vi "poly_h5_write_array_1d_DBL.vi"(0 "h5 dir ref":i32, 1 "dataset name":string, 5 "array":dbl[](array[numeric]), 7 "units (au)":string="au", 11 "error in (no error)":errorcluster, 12 "dim (index)":string="index") -> (4 "h5 obj ref":i32, 15 "error out":errorcluster)   [LabVIEW 2015]
uses:
  <vilib>/addons/h5labview2/base/lib_path.vi
  <vilib>/addons/h5labview2/base/H5Equery.vi
  <vilib>/addons/h5labview2/dataset/H5Dwrite.llb/H5Dwrite.xnode
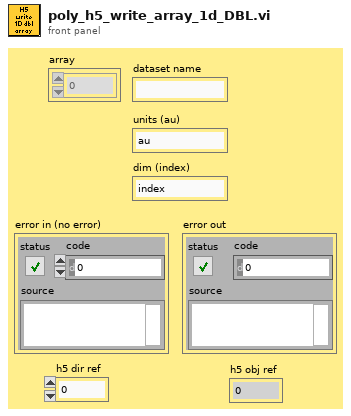
[diagram p1: front panel]
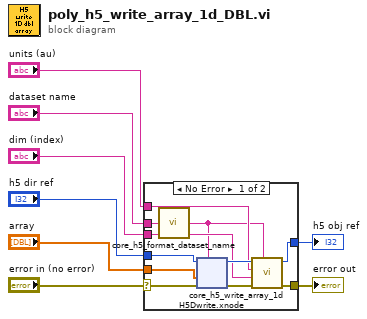
[diagram p0: block diagram]
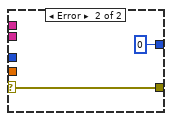
[diagram p2: hidden frame]
diagram:
  n1 = case shown="No Error" "error in (no error)" {
    selector: "error in (no error)" -> [w17 w40]
    tunnel: "h5 dir ref" -> [w19 _]
    tunnel: "array" -> [w18 _]
    tunnel: "dataset name" -> [w10 _]
    tunnel: [w13 w40] -> w6
    tunnel: [w15 0] -> w5
    tunnel: "dim (index)" -> [w12 _]
    tunnel: "units (au)" -> [w11 _]
    frame No Error {
      n2 = call "core_h5_format_dataset_name.vi"("dataset name in"=w10) -> ("dataset name out"=w9:string)  [unwired: 8 in]
      n3 = xnode "H5Dwrite.xnode"("dataset name"=w9, "error in (no error)"=w17, "data"=w18, "ref in"=w19) -> ("error out"=w14:errorcluster, "ref out"=w16:i32)  [unwired: 3 in, 1 out]
      n4 = call "core_h5_write_array_1d.vi"("dataset name"=w9, "error in (no error)"=w14, "dim (index)"=w12, "units (au)"=w11, "h5 obj ref"=w16) -> ("error out"=w13:errorcluster, "h5 obj ref"=w15:i32)  [unwired: 5 in]
    }
    frame Error {
    }
  }
  "error out" <- w6
  "h5 obj ref" <- w5
